vi "总磷总氮MB_api.vi"(6 "Slave ID":u8=1, 7 "STEP":enum16{"open", "read", "write", "close"}(ring)=enum."read", 8 "Error in":errorcluster caption="Error in (no error)", 9 "values":u16[](array[numeric]), 10 "quantity":u16, 11 "starting address":u16 format="%04xH") -> (0 "error out":errorcluster, 1 "MB session out":refnum<class "MB_Master.lvclass">, 2 "MB_TCP session":refnum<class "MB_Master_TCP.lvclass">, 3 "Registers":u16[](array[numeric]))   [LabVIEW 2016, in "斯坦道总磷总氮.lvlib"]
uses:
  <vilib>/Plasmionique/MB Master/MB_Master/MB_Master.lvclass
  <vilib>/Plasmionique/MB Master/MB_Master_TCP/MB_Master_TCP.lvclass
  C:/Program Files (x86)/National Instruments/LabVIEW 2016/vi.lib/Plasmionique/MB Master/MB_Master/MB_Master.lvclass
  <vilib>/Plasmionique/MB Master/MB_Master_Serial/MB_Master_Serial.lvclass
  <vilib>/Plasmionique/MB Master/MB Master.lvlib
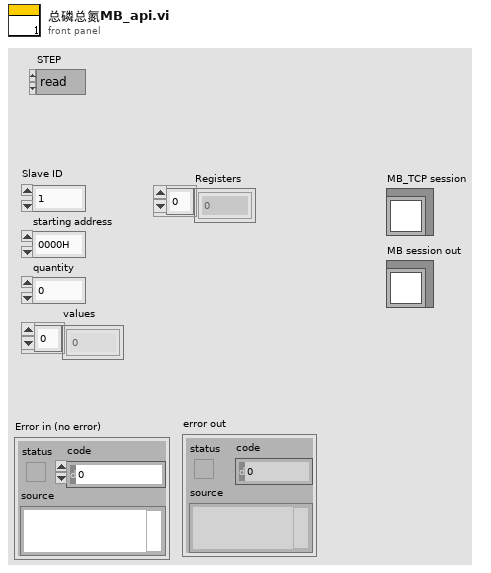
[diagram p1: front panel]
types:
  T1 = cluster{"baud rate (bps)":u32, "stop bits":u16, "parity":u16, "flow control":u16, "timeout":u32, "retries":i32}
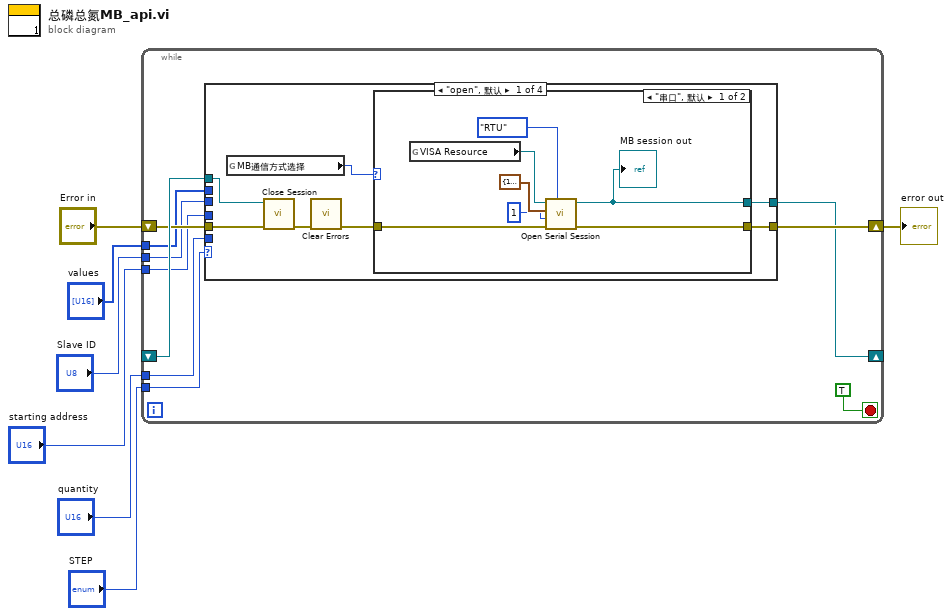
[diagram p0: block diagram]
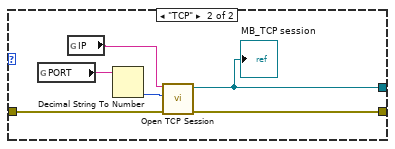
[diagram p2: hidden frame]
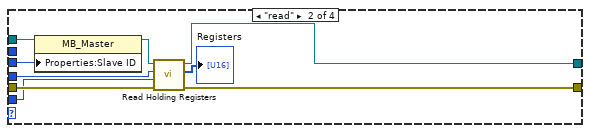
[diagram p3: hidden frame]
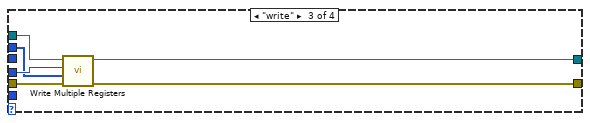
[diagram p4: hidden frame]
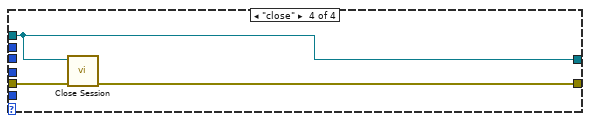
[diagram p5: hidden frame]
diagram:
  n1 = while {
    shift-right: [w8] -> _
    shift-left: _ -> [w17]
    shift-right: [w9] -> w6
    shift-left: "Error in" -> [w16]
    tunnel: "Slave ID" -> [w15]
    tunnel: "starting address" -> [w14]
    tunnel: "quantity" -> [w13]
    tunnel: "STEP" -> [w12]
    tunnel: "values" -> [w11]
    stop <- TRUE stop-if-true
    n2 = case shown="\"open\", 默认" w12 {
      tunnel: w17 -> [w22 w39 w50 w53]
      tunnel: w16 -> [w21 w46 w52 w55]
      tunnel: [w23 w45 w49 w53] -> w8
      tunnel: [w24 w44 w51 w54] -> w9
      tunnel: w15 -> [_ w42 _ _]
      tunnel: w14 -> [_ w41 w48 _]
      tunnel: w13 -> [_ w40 _ _]
      tunnel: w11 -> [_ _ w47 _]
      frame "open", Default {
        n3 = global read "总磷总氮断电保存全局变量.vi" "MB通信方式选择"() -> (w20:enum16{"串口", "TCP"})
        n4 = call-dynamic "Close Session.vi"("error in (no error)"=w21, "MB session in"=w22) -> ("error out"=w19:errorcluster)  [unwired: 9 in]
        n5 = call <vilib>:"Clear Errors.vi"("error in (no error)"=w19) -> ("error out"=w18:errorcluster)  [unwired: 5 in, 1 out]
        n6 = case shown="\"串口\", 默认" w20 {
          tunnel: [w29 w35] -> w24
          tunnel: [w25 w34] -> w23
          tunnel: w18 -> [w27 w36]
          frame "串口", Default {
            n7 = global read "总磷总氮断电保存全局变量.vi" "VISA Resource"() -> (w26:refnum<visa-resource-name>)
            n8 = call <vilib>:"Open Serial Session.vi"("Mode (RTU)"=enum16{"RTU", "ASCII"}."RTU", "Error in"=w27, "Slave ID"=u8 1, "Serial Config"=T1 {"baud rate (bps)"=115200, "stop bits"=10, "parity"=0, "flow control"=0, "timeout"=500, "retries"=1}, "VISA Resource"=w26) -> ("Error out"=w29:errorcluster, "MB_Serial session"=w25:refnum<class "MB_Master_Serial.lvclass">)  [unwired: 5 in]
            "MB session out" <- w25
          }
          frame "TCP" {
            n9 = global read "总磷总氮断电保存全局变量.vi" "PORT"() -> (w33:string)
            n10 = global read "总磷总氮断电保存全局变量.vi" "IP"() -> (w32:string)
            n11 = Decimal String To Number(string=w33) -> (number=w37:i32)  [unwired: 2 in, 1 out]
            n12 = call <vilib>:"Open TCP Session.vi"("error in (no error)"=w36, "Port (502)"=w37, "IP Address"=w32) -> ("error out"=w35:errorcluster, "MB_TCP session"=w34:refnum<class "MB_Master_TCP.lvclass">)  [unwired: 7 in]
            "MB_TCP session" <- w34
          }
        }
      }
      frame "read" {
        n13 = property class="MB_Master"(reference=w39, "Properties:Slave ID"=w42) -> (reference out=w38:refnum<class "MB_Master.lvclass">)  [unwired: 1 in, 1 out]
        n14 = call <vilib>:"Read Holding Registers.vi"("error in (no error)"=w46, "quantity"=w40, "starting address"=w41, "MB session in"=w38) -> ("error out"=w44:errorcluster, "Registers"=→"Registers":u16[], "MB session out"=w45:refnum<class "MB_Master.lvclass">)  [unwired: 5 in]
      }
      frame "write" {
        n15 = call <vilib>:"Write Multiple Registers.vi"("error in (no error)"=w52, "values"=w47, "starting address"=w48, "MB session in"=w50) -> ("error out"=w51:errorcluster, "MB session out"=w49:refnum<class "MB_Master.lvclass">)  [unwired: 6 in]
      }
      frame "close" {
        n16 = call-dynamic "Close Session.vi"("error in (no error)"=w55, "MB session in"=w53) -> ("error out"=w54:errorcluster)  [unwired: 9 in]
      }
    }
  }
  "error out" <- w6
